vi "McP789A-Move-v0.80.vi"(4 "Initializing MCP":bool=TRUE, 5 "Change Counter Position Manually":bool, 6 "error in":errorcluster, 8 "New Wavelength (nm)":dbl=600.0 min=0.0 max=100000.0 format="%.3f", 9 "Grating Density":enum16{"150", "300", "600", "1200", "1800"}(ring)=enum."1800") -> (0 "error out":errorcluster={"status"=TRUE, "code"=65, "source"="McP Timeout"}, 1 "Final Stepper Position":i32=-1000000, 2 "Final Wavelenth (nm)":dbl=222.0 format="%.2f", 3 "Final CounterReading":dbl=10000.0 min=0.0 max=26000.0 format="%.2f")   [LabVIEW 2020]
doc: "McPherson 789A-3 controller Vi to control McPherson 2075 spectrometer through serial port. If running directly, you need to initialize the serial port and the spectrometer. During this process, if the scan velocity returns to be 0, the program is suspended. You need to change the velocity manually to unblock."
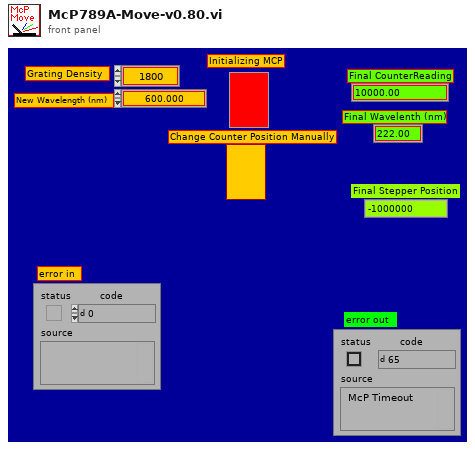
[diagram p1: front panel]
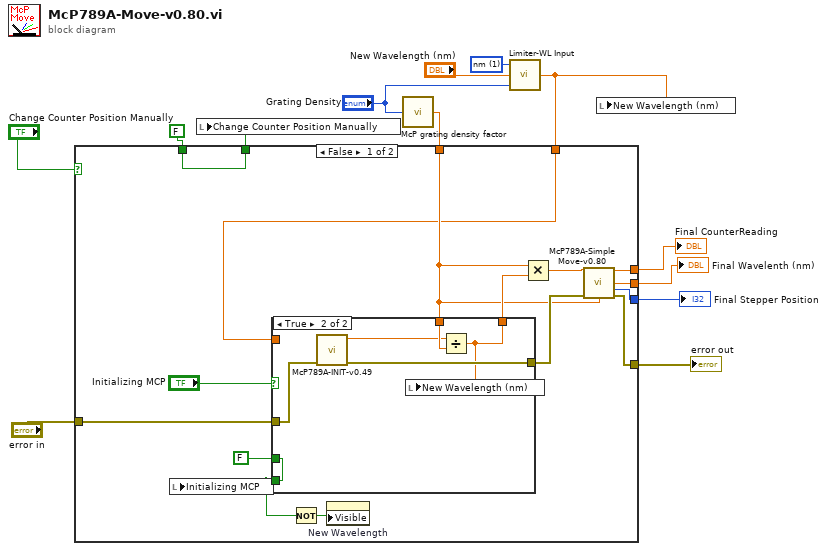
[diagram p0: block diagram]
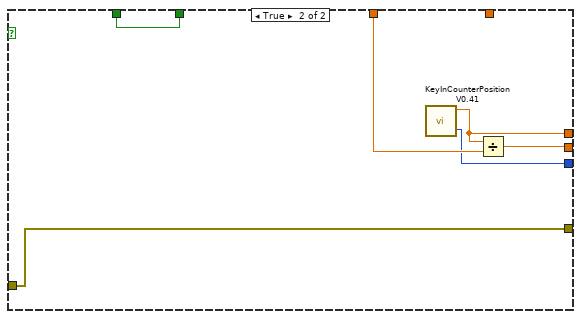
[diagram p3: hidden frame]
diagram:
  w4 = 1 items=["Point #", "nm", "eV", "meV", "cm-1"] ("X-Axis")
  n1 = call "McP grating density factor.vi"("Grating Density"="Grating Density") -> ("GratingFactor"=w1:dbl)
  n2 = call "Limiter-WL Input.vi"("Current Grating Density"="Grating Density", "Central WL Input"="New Wavelength (nm)", "X-Axis"=w4) -> ("Central WL output"=w3:dbl)
  n3 = case shown="False" "Change Counter Position Manually" {
    tunnel: [w27 w40] -> w13
    tunnel: [w25 w41] -> w12
    tunnel: [w24 w42] -> w11
    tunnel: "error in" -> [w23 w42]
    tunnel: w1 -> [w16 w39]
    tunnel: [w21 w43] -> w8
    tunnel: FALSE -> [w21 w43]
    tunnel: [w15 w38] -> w6
    tunnel: w3 -> [w14 _]
    frame False {
      n4 = case shown="True" "Initializing MCP" {
        tunnel: w23 -> [w31 w33]
        tunnel: [w31 w37] -> w28
        tunnel: w16 -> [_ w36]
        tunnel: [w30 w35] -> w26
        tunnel: w14 -> [w30 _]
        tunnel: [w29 w34] -> w18
        tunnel: FALSE -> [w29 w34]
        frame False {
        }
        frame True {
          n5 = call "McP789A-INIT-v0.49.vi"("error in (no error)"=w33) -> ("error out"=w37:errorcluster, "MCP CounterReading"=w32:dbl)  [unwired: 4 in, 2 out]
          n6 = Divide(x=w32, y=w36) -> (x/y=w35:dbl)
          n7 = local write "New Wavelength (nm)"(w35) -> ()
        }
      }
      n8 = local write "Initializing MCP"(w18) -> ()
      n9 = Not(x=w18) -> (.not. x?=w19:bool)
      n10 = property on="New Wavelength" class="DigNum (strict)"("Visible"=w19) -> ()  [unwired: 2 in, 2 out]
      n11 = Multiply(x=w16, y=w26) -> (x*y=w17:dbl)
      n12 = call "McP789A-SimpleMove-v0.80.vi"("New Counter Position"=w17, "error in (no error)"=w28, "Grating factor"=w16) -> ("Final CounterRdg"=w27:dbl, "Final Wavelenth(nm)"=w25:dbl, "Final Stepper Position"=w15:i32, "error out"=w24:errorcluster)  [unwired: 9 in]
    }
    frame True {
      n13 = call "KeyInCounterPosition V0.41.vi"() -> ("Counter Position output"=w40:dbl, "Stepper Position"=w38:i32)  [unwired: 1 in]
      n14 = Divide(x=w40, y=w39) -> (x/y=w41:dbl)
    }
  }
  "Final Wavelenth (nm)" <- w12
  "Final CounterReading" <- w13
  "error out" <- w11
  "Final Stepper Position" <- w6
  n15 = local write "Change Counter Position Manually"(w8) -> ()
  n16 = local write "New Wavelength (nm)"(w3) -> ()
